vi "GetTextInformation.vi"(8 "error in (no error)":errorcluster, 10 "Input":string, 11 "EAN-13 in":refnum<class "EAN-13.lvclass">) -> (0 "error out":errorcluster, 1 "Text":string, 2 "Text Positions":T1[](array[typedef]), 3 "EAN-13 out":refnum<class "EAN-13.lvclass">)   [LabVIEW 2013, in "BarCodes.lvlib" / "EAN-13.lvclass"]
doc: "Returns an array of clusters describing how text will be sized and positioned and the actual text to place below the bar code. The Start Index is the index in the returned string that each text info entry refers to. The length is the number of characters in the returned string that each text info entry refers to. The Text Rectangle is the rectangle to draw text in. The Clearing Rectangle is the rectangle to paint with the barcode's light color to make the text clear and visible. The font information is passed into the text writing function."
uses:
  EAN-13.lvclass
  BarCode/TextPosition.ctl
  BarCode/BarCode.lvclass
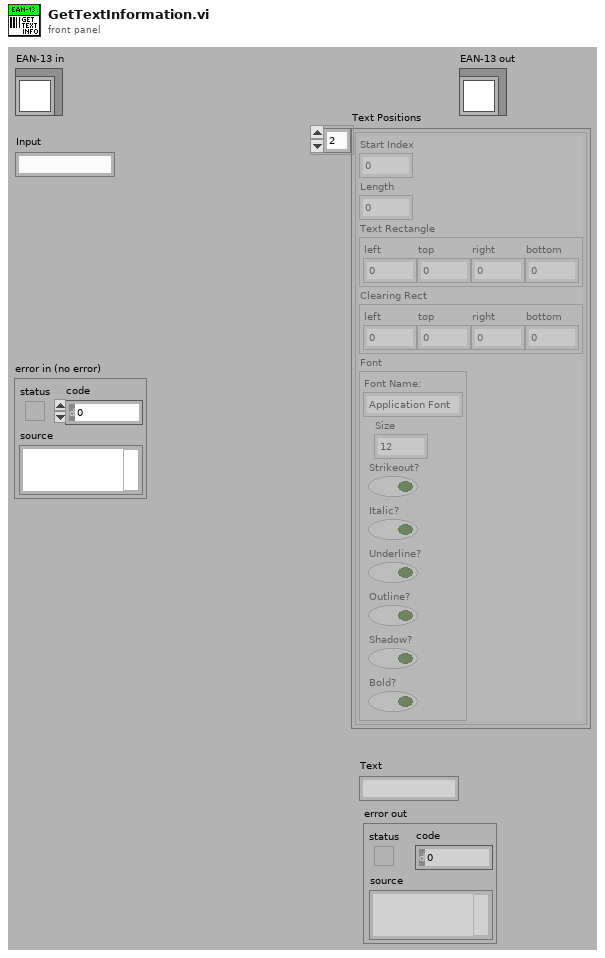
[diagram p1: front panel]
types:
  T1 = typedef "BarCodes.lvlib/BarCode.lvclass/TextPosition.ctl" = cluster{"Start Index":u8, "Length":u8, "Text Rectangle":cluster{"left":i16, "top":i16, "right":i16, "bottom":i16}, "Clearing Rect":cluster{"left":i16, "top":i16, "right":i16, "bottom":i16}, "Font":cluster{"Font Name:":string, "Size":i16, "Strikeout?":bool, "Italic?":bool, "Underline?":bool, "Outline?":bool, "Shadow?":bool, "Bold?":bool}}
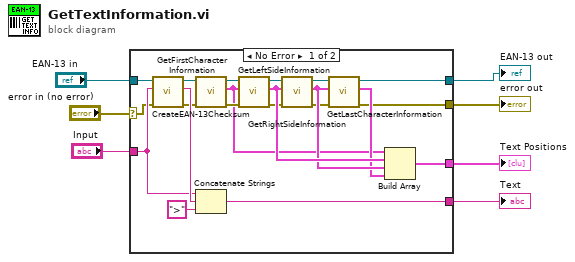
[diagram p0: block diagram]
diagram:
  n1 = case shown="No Error" "error in (no error)" {
    selector: "error in (no error)" -> [w15 w29]
    tunnel: "Input" -> [w26 _]
    tunnel: "EAN-13 in" -> [w22 w30]
    tunnel: [w17 _] -> w5
    tunnel: [w16 w30] -> w4
    tunnel: [w10 w29] -> w2
    tunnel: [w9 _] -> w1
    frame No Error {
      n2 = call "CreateEAN-13Checksum.vi"("error in (no error)"=w15, "String"=w26, "EAN-13 in"=w22) -> ("error out"=w14:errorcluster, "Checksum"=w28:string, "EAN-13 out"=w23:refnum<class "EAN-13.lvclass">)  [unwired: 6 in]
      n3 = call-dynamic "GetFirstCharacterInformation.vi"("error in (no error)"=w14, "EAN-13 In"=w23) -> ("error out"=w13:errorcluster, "Text Information"=w8:T1, "EAN-13 out"=w24:refnum<class "EAN-13.lvclass">)  [unwired: 7 in]
      n4 = Concatenate Strings(w26, w28, ">" ("string")) -> (w9:string)
      n5 = call-dynamic "GetLeftSideInformation.vi"("error in (no error)"=w13, "FirstCharInfo"=w8, "EAN in"=w24) -> ("error out"=w12:errorcluster, "Text Position"=w27:T1, "EAN out"=w25:refnum<class "EAN-13.lvclass">)  [unwired: 6 in]
      n6 = call "GetRightSideInformation.vi"("error in (no error)"=w12, "Left position"=w27, "EAN-13 in"=w25) -> ("error out"=w11:errorcluster, "Right text position"=w20:T1, "EAN-13 out"=w21:refnum<class "EAN-13.lvclass">)  [unwired: 6 in]
      n7 = call-dynamic "GetLastCharacterInformation.vi"("error in (no error)"=w11, "Right Text Information"=w20, "EAN-13 In"=w21) -> ("error out"=w10:errorcluster, "Text Information"=w19:T1, "EAN-13 out"=w16:refnum<class "EAN-13.lvclass">)  [unwired: 6 in]
      n8 = Build Array(w8, w27, w20, w19) -> (w17:T1[])
    }
    frame Error {
    }
  }
  "error out" <- w2
  "EAN-13 out" <- w4
  "Text Positions" <- w5
  "Text" <- w1
